vi "RampVoltage.vi"() -> ()   [LabVIEW 2016]
uses:
  <vilib>/DAQmx/write.llb/DAQmx Write (Analog 2D DBL NChan NSamp).vi
  <vilib>/DAQmx/create/channels.llb/DAQmx Create Channel (AO-Voltage-Basic).vi
  <vilib>/DAQmx/configure/timing.llb/DAQmx Timing (Sample Clock).vi
  <vilib>/DAQmx/configure/trigger.llb/DAQmx Start Trigger (Digital Edge).vi
  <vilib>/DAQmx/miscellaneous.llb/DAQmx Fill In Error Info.vi
  <resource>/objmgr/daqmx.rc
panel:
  in  "Ramp duration (ms)":dbl
  out "appended array 2":dbl[][](array[numeric])
  in  "No of samples in ramp":dbl
  in  "Ramp Amplitude (V)}":dbl
  in  "error in":errorcluster
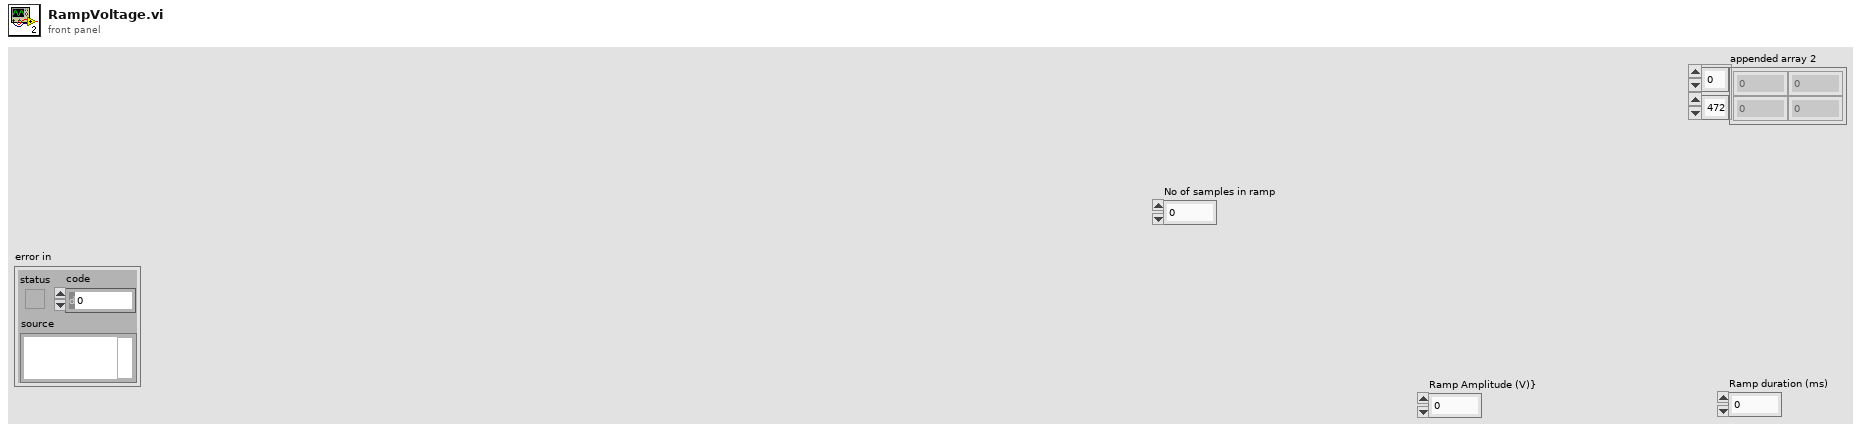
[diagram p1: front panel]
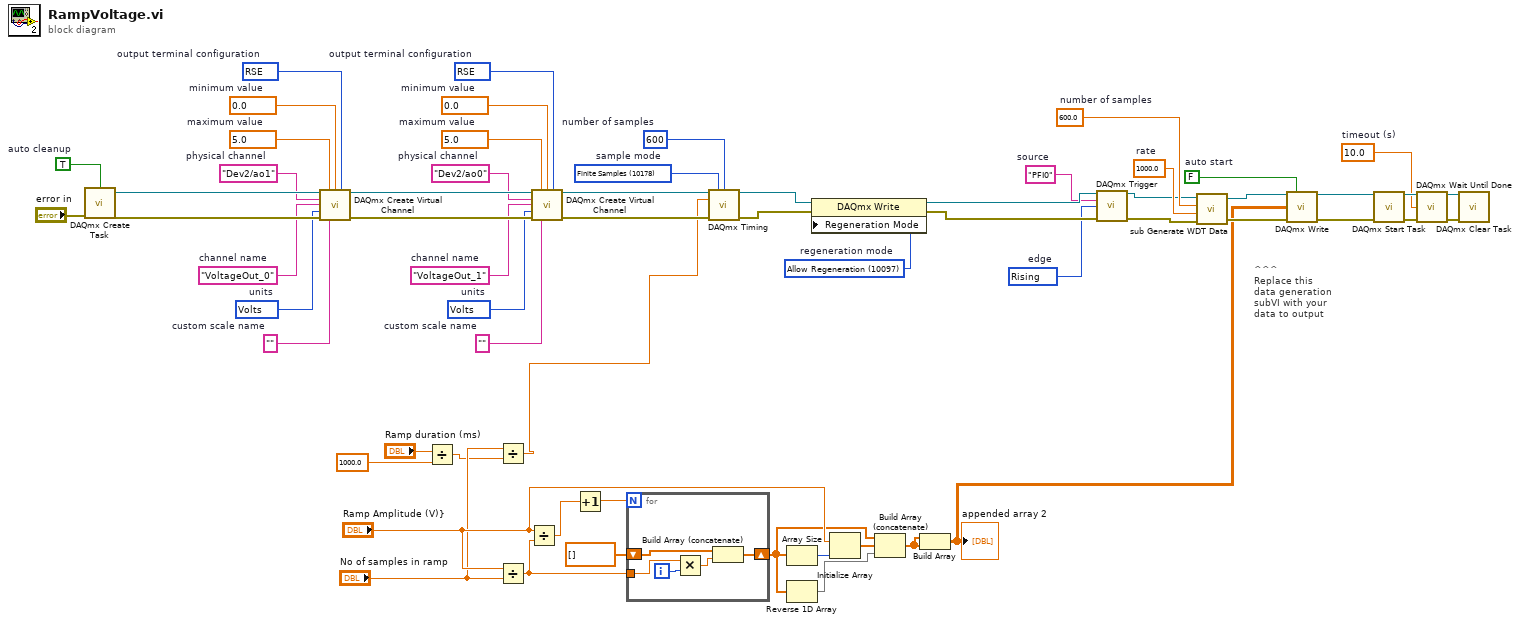
[diagram p0: block diagram]
diagram:
  w19 = 10280 items=["Rising"=10280, "Falling"=10171]  # edge
  w20 = "PFI0"  # source
  w22 = 10097 items=["Allow Regeneration"=10097, "Do Not Allow Regeneration"=10158]  # regeneration mode
  w25 = 10178 items=["Finite Samples"=10178, "Continuous Samples"=10123, "Hardware Timed Single Point"=12522]  # sample mode
  w26 = 600  # number of samples
  w29 = 10083 items=["Default"=-1, "RSE"=10083, "Differential"=10106, "Pseudodifferential"=12529]  # output terminal configuration
  w30 = 10348 items=["Volts"=10348, "From Custom Scale"=10065]  # units
  w31 = "VoltageOut_1"  # channel name
  w33 = ""  # custom scale name
  w34 = 0.0  # minimum value
  w35 = 5.0  # maximum value
  w36 = "Dev2/ao0"  # physical channel
  w38 = 10083 items=["Default"=-1, "RSE"=10083, "Differential"=10106, "Pseudodifferential"=12529]  # output terminal configuration
  w39 = 10348 items=["Volts"=10348, "From Custom Scale"=10065]  # units
  w40 = "VoltageOut_0"  # channel name
  w42 = ""  # custom scale name
  w43 = 0.0  # minimum value
  w44 = 5.0  # maximum value
  w45 = "Dev2/ao1"  # physical channel
  w47 = TRUE  # auto cleanup
  w53 = 10.0  # timeout (s)
  w57 = 1000.0  # rate
  w58 = 600.0  # number of samples
  w61 = FALSE  # auto start
  # "^^^\nReplace this\ndata generation\nsubVI with your\ndata to output"
  n1 = call <vilib>:"DAQmx Create Task.vi"("auto cleanup"=w47, "error in"="error in") -> ("task out"=w46:refnum<k21>, "error out"=w48:errorcluster)  [unwired: 12 in]
  n2 = call-poly <vilib>:"DAQmx Create Virtual Channel.vi"("task in"=w46, "maximum value"=w44, "minimum value"=w43, "output terminal configuration"=w38, "physical channels"=w45, "name to assign"=w40, "units"=w39, "error in"=w48, "custom scale name"=w42) -> ("task out"=w37:refnum<k21>, "error out"=w41:errorcluster)  [unwired: 5 in]
  n3 = Divide(x="Ramp duration (ms)", y=1000.0) -> (x/y=w2:dbl)
  n4 = Divide(x="No of samples in ramp", y=w2) -> (x/y=w1:dbl)
  n5 = Divide(x="Ramp Amplitude (V)}", y="No of samples in ramp") -> (x/y=w15:dbl)
  n6 = Divide(x="Ramp Amplitude (V)}", y=w15) -> (x/y=w14:dbl)
  n7 = call-poly <vilib>:"DAQmx Create Virtual Channel.vi"("task in"=w37, "maximum value"=w35, "minimum value"=w34, "output terminal configuration"=w29, "physical channels"=w36, "name to assign"=w31, "units"=w30, "error in"=w41, "custom scale name"=w33) -> ("task out"=w27:refnum<k21>, "error out"=w32:errorcluster)  [unwired: 5 in]
  n8 = Increment(x=w14) -> (x+1=w13:dbl)
  n9 = for {
    N: w13 -> [_]
    shift-right: [w64] -> w10
    shift-left: dbl[] [] -> [w63]
    tunnel: w15 -> [w62]
    i -> [w66]
    n10 = Multiply(x=w62, y=w66) -> (x*y=w65:dbl)
    n11 = Build Array (concatenate)(w63, w65) -> (w64:dbl[])
  }
  n12 = call-poly <vilib>:"DAQmx Timing.vi"("task/channels in"=w27, "sample mode"=w25, "samples per channel"=w26, "rate"=w1, "error in"=w32) -> ("task out"=w24:refnum<k21>, "error out"=w28:errorcluster)  [unwired: 9 in]
  n13 = Array Size(array=w10) -> (size(s)=w11:i32)
  n14 = Reverse 1D Array(array=w10) -> (reversed array=w8:dbl[])
  n15 = property class="DAQmx Write"(reference=w24, error in=w28, "Regeneration Mode"=w22) -> (reference out=w21:refnum<k21>, error out=w23:errorcluster)
  n16 = Initialize Array("Ramp Amplitude (V)}", w11) -> (w9:dbl[])
  n17 = Build Array (concatenate)(w10, w9, w8) -> (w7:dbl[])
  n18 = Build Array(w7, w7) -> (w6:dbl[][])
  "appended array 2" <- w6
  n19 = call-poly <vilib>:"DAQmx Trigger.vi"("task/channels in"=w21, "source"=w20, "edge"=w19, "error in"=w23) -> ("task out"=w18:refnum<k21>, "error out"=w17:errorcluster)  [unwired: 10 in]
  n20 = call <vilib>:"sub Generate WDT Data.vi"("task in"=w18, "number of samples"=w58, "update rate"=w57, "error in"=w17) -> ("task out"=w59:refnum<k21>, "error out"=w60:errorcluster)  [unwired: 1 in, 1 out]
  n21 = call-poly <vilib>:"DAQmx Write.vi"("task/channels in"=w59, "auto start"=w61, "data"=w6, "error in"=w60) -> ("task out"=w52:refnum<k21>, "error out"=w51:errorcluster)  [unwired: 9 in, 1 out]
  n22 = call <vilib>:"DAQmx Start Task.vi"("task/channels in"=w52, "error in"=w51) -> ("task out"=w56:refnum<k21>, "error out"=w55:errorcluster)  [unwired: 12 in]
  n23 = call <vilib>:"DAQmx Wait Until Done.vi"("task/channels in"=w56, "timeout (sec)"=w53, "error in"=w55) -> ("task out"=w50:refnum<k21>, "error out"=w54:errorcluster)  [unwired: 11 in]
  n24 = call <vilib>:"DAQmx Clear Task.vi"("task in"=w50, "error in"=w54) -> ()  [unwired: 13 in, 1 out]
